vi "UIRefs BPG Waveform.vi"(8 "error in (no error)":errorcluster, 11 "BPG in":refnum<class "BPG.lvclass">) -> (0 "error out":errorcluster, 3 "BPG out":refnum<class "BPG.lvclass">)   [LabVIEW 2021]
uses:
  BPG.lvclass
  BPG.lvclass/BPG.ctl
  C:/Program Files/National Instruments/LabVIEW 2021/vi.lib/MGI/Panel Manager/Panel Actor/Panel Actor/Panel Actor.lvclass
  C:/Program Files/National Instruments/LabVIEW 2021/vi.lib/ActorFramework/Actor/Actor.lvclass
  C:/PPLs/BPG/BPG/BPG.lvclass
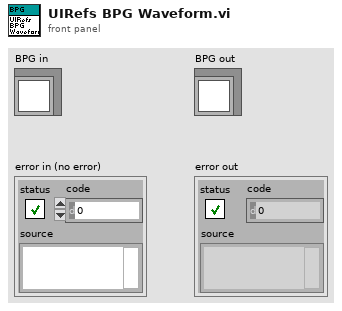
[diagram p1: front panel]
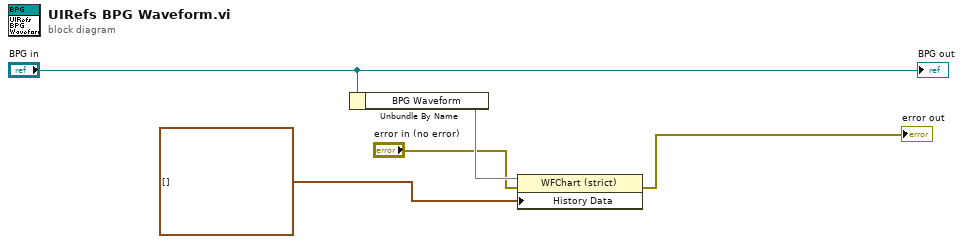
[diagram p0: block diagram]
diagram:
  n1 = Unbundle By Name("BPG in") -> ("BPG Waveform"=w4)
  n2 = property class="WFChart (strict)"(reference=w4, error in="error in (no error)", "History Data"=waveform(dbl)[] []) -> (error out=→"error out":errorcluster)  [unwired: 1 out]
  "BPG out" <- "BPG in"
